vi "Write_data.vi"(0 "DVR In":refnum<data-value>, 5 "DATA":T1, 7 "Name":string, 11 "error in":errorcluster) -> (4 "DVR Out":refnum<data-value>, 15 "error out":errorcluster)   [LabVIEW 2020, in "Communication.lvclass"]
doc: "Write data to notifier."
uses:
  Classes/Communication/Communication.lvclass
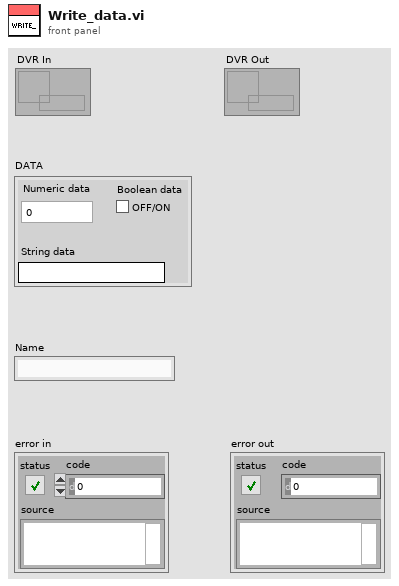
[diagram p1: front panel]
types:
  T1 = cluster{"Numeric data":dbl, "String data":string, "Boolean data":bool}
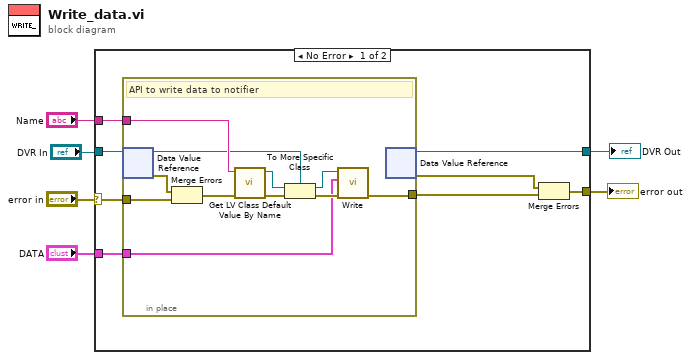
[diagram p0: block diagram]
diagram:
  n1 = case shown="No Error" "error in" {
    selector: "error in" -> [w14 w26]
    tunnel: "DVR In" -> [w8 w27]
    tunnel: "DATA" -> [w13 _]
    tunnel: [w11 w26] -> w4
    tunnel: [w7 w27] -> w1
    tunnel: "Name" -> [w10 _]
    frame No Error {
      n2 = in-place {
        in-place-border: w14 -> [w24]
        in-place-border: w13 -> [w15]
        in-place-border: w10 -> [w21]
        in-place-border: [w18] -> w9
        # "API to write data to notifier"
        n3 = in-place-dvr #1(w8) -> (w19:refnum<class "Communication.lvclass">, w25:errorcluster)
        n4 = Merge Errors(w25, w24) -> (w22:errorcluster)
        n5 = call <vilib>:"Get LV Class Default Value By Name.vi"("error in (no error)"=w22, "class name"=w21) -> ("error out"=w23:errorcluster, "object"=w20:refnum<class>)  [unwired: 8 in]
        n6 = To More Specific Class(target class=w19, reference=w20, error in=w23) -> (specific class reference=w16:refnum<class "Communication.lvclass">, error out=w17:errorcluster)
        n7 = call-dynamic "Write.vi"("error in (no error)"=w17, "DATA"=w15, "Communication in"=w16) -> ("error out"=w18:errorcluster)  [unwired: 7 in, 1 out]
        n8 = in-place-dvr #1() -> (w7:refnum<data-value>, w12:errorcluster)  [unwired: 1 in]
      }
      n9 = Merge Errors(w12, w9) -> (w11:errorcluster)
    }
    frame Error {
    }
  }
  "error out" <- w4
  "DVR Out" <- w1
